vi "Target_side_DAQ_data.vi"() -> ()   [LabVIEW 2017]
panel:
  in  "Boolean":bool
  out "String":string
  in  "stop":bool
  out "Waveform Chart":waveform(i32)(graph)
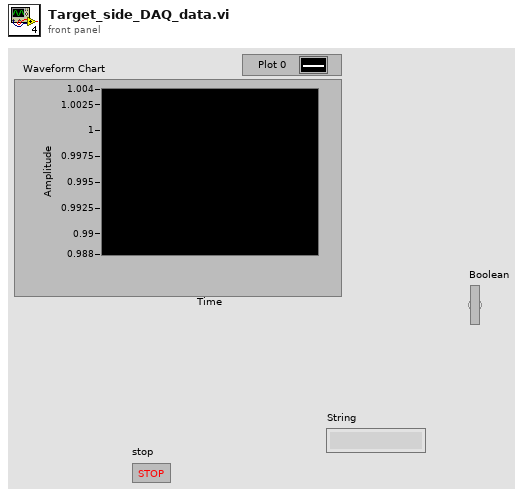
[diagram p1: front panel]
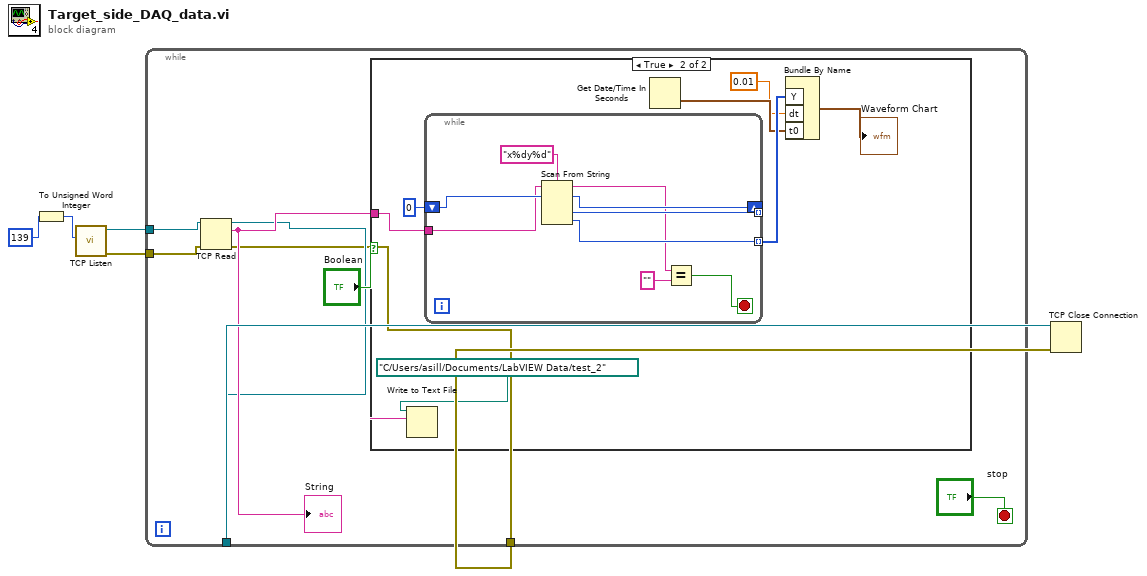
[diagram p0: block diagram]
diagram:
  n1 = To Unsigned Word Integer(number=139) -> (unsigned 16bit integer=w1:u16)
  n2 = call <vilib>:"TCP Listen.vi"("port"=w1) -> ("error out"=w5:errorcluster, "connection ID"=w6:refnum<k5>)  [unwired: 6 in, 3 out]
  n3 = while {
    tunnel: w6 -> [w13]
    tunnel: w5 -> [w12]
    tunnel: [w7] -> w4
    tunnel: [w8] -> w3
    stop <- "stop" stop-if-true
    n4 = TCP Read(connection ID=w13, error in (no error)=w12) -> (connection ID out=w8:refnum<k5>, data out=w10:string, error out=w7:errorcluster)  [unwired: 3 in]
    "String" <- w10
    n5 = case shown="True" "Boolean" {
      tunnel: w10 -> [_ w15]
      frame False {
      }
      frame True {
        n6 = Write to Text File(file (use dialog)=path "C:/Users/asill/Documents/LabVIEW Data/test_2", text=w15) -> ()  [unwired: 2 in, 3 out]
        n7 = while {
          tunnel: [w28] -> _ mode=indexing
          tunnel: [w27] -> w19 mode=indexing
          shift-right: [w26] -> _
          shift-left: u32 0 -> [w25]
          tunnel: w15 -> [w21]
          stop <- w24 stop-if-true
          n8 = Scan From String(format string="x%dy%d", input string=w21, initial scan location=w25) -> (remaining string=w23:string, offset past scan=w26:u32, output 1=w28:i32, output 2=w27:i32)  [unwired: 3 in, 1 out]
          n9 = Equal?(x=w23, y="") -> (x = y?=w24:bool)
        }
        n10 = Get Date/Time In Seconds() -> (seconds since 1Jan1904=w17:timestamp)
        n11 = Bundle By Name("Y"=w19, "dt"=0.01, "t0"=w17) -> (→"Waveform Chart":waveform(i32))  [unwired: 1 in]
      }
    }
  }
  n12 = TCP Close Connection(connection ID=w3, error in (no error)=w4) -> ()  [unwired: 1 in, 2 out]
